vi "core_h5_write_array_2d.vi"(6 "dim2 (index)":string="index", 7 "dataset name":string, 8 "error in (no error)":errorcluster, 9 "dim1 (index)":string="index", 10 "units (au)":string="au", 11 "h5 obj ref":i32) -> (0 "error out":errorcluster, 3 "h5 obj ref":i32)   [LabVIEW 2015]
uses:
  <vilib>/addons/h5labview2/base/lib_path.vi
  <vilib>/addons/h5labview2/base/H5Equery.vi
  <vilib>/addons/h5labview2/attrib/H5Awrite.llb/H5Awrite.xnode
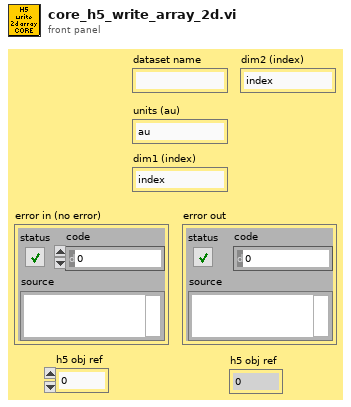
[diagram p1: front panel]
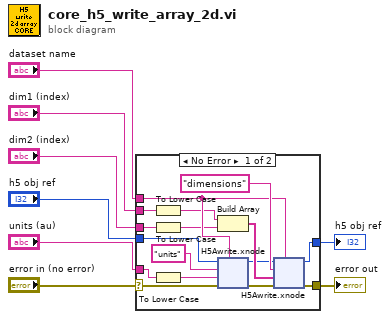
[diagram p0: block diagram]
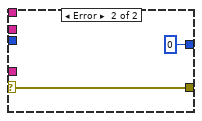
[diagram p2: hidden frame]
diagram:
  n1 = case shown="No Error" "error in (no error)" {
    selector: "error in (no error)" -> [w15 w64]
    tunnel: "h5 obj ref" -> [w16 _]
    tunnel: "dataset name" -> [w19 _]
    tunnel: [w18 w64] -> w7
    tunnel: [w17 0] -> w6
    tunnel: "dim1 (index)" -> [w14 _]
    tunnel: "dim2 (index)" -> [w12 _]
    tunnel: "units (au)" -> [w10 _]
    frame No Error {
      n2 = To Lower Case(string=w14) -> (all lower case string=w13:string)
      n3 = To Lower Case(string=w12) -> (all lower case string=w11:string)
      n4 = To Lower Case(string=w10) -> (all lower case string=w9:string)
      n5 = Build Array(w13, w11) -> (w22:string[])
      n6 = xnode "H5Awrite.xnode"("object name"=w19, "error in (no error)"=w15, "data"=w9, "attrib name"="units", "ref in"=w16) -> ("error out"=w21:errorcluster, "ref out"=w20:i32)  [unwired: 2 in, 1 out]
      n7 = xnode "H5Awrite.xnode"("object name"=w19, "error in (no error)"=w21, "data"=w22, "attrib name"="dimensions", "ref in"=w20) -> ("error out"=w18:errorcluster, "ref out"=w17:i32)  [unwired: 2 in, 1 out]
    }
    frame Error {
    }
  }
  "error out" <- w7
  "h5 obj ref" <- w6
